vi "TempMonitor.vi"() -> (1 "Temp Out of Range":bool, 3 "Waveform Chart":waveform(dbl)(graph))   [LabVIEW 2013]
panel:
  in  "Min Temp":dbl=15.0
  in  "Max Temp":dbl=30.0
  out "Ch32":dbl
  out "Ch31":dbl
  out "Ch30":dbl
  out "Ch29":dbl
  out "Ch28":dbl
  out "Ch27":dbl
  out "Ch26":dbl
  out "Ch25":dbl
  out "Ch24":dbl
  out "Ch23":dbl
  out "Ch22":dbl
  out "Ch21":dbl
  out "Ch20":dbl
  out "Ch19":dbl
  out "Ch18":dbl
  out "Ch17":dbl
  in  "stop":bool
  out "Ch16":dbl
  out "Ch15":dbl
  out "Ch14":dbl
  out "Ch13":dbl
  out "Ch12":dbl
  out "Ch11":dbl
  out "Ch10":dbl
  out "Ch9":dbl
  out "Ch8":dbl
  out "Ch7":dbl
  out "Ch6":dbl
  out "Ch5":dbl
  out "Ch4":dbl
  out "Ch3":dbl
  out "Ch2":dbl
  out "Ch1":dbl
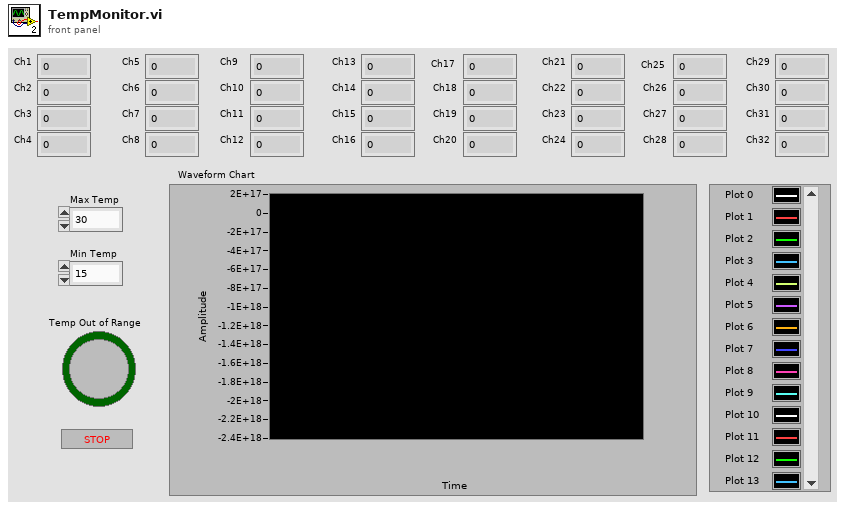
[diagram p1: front panel]
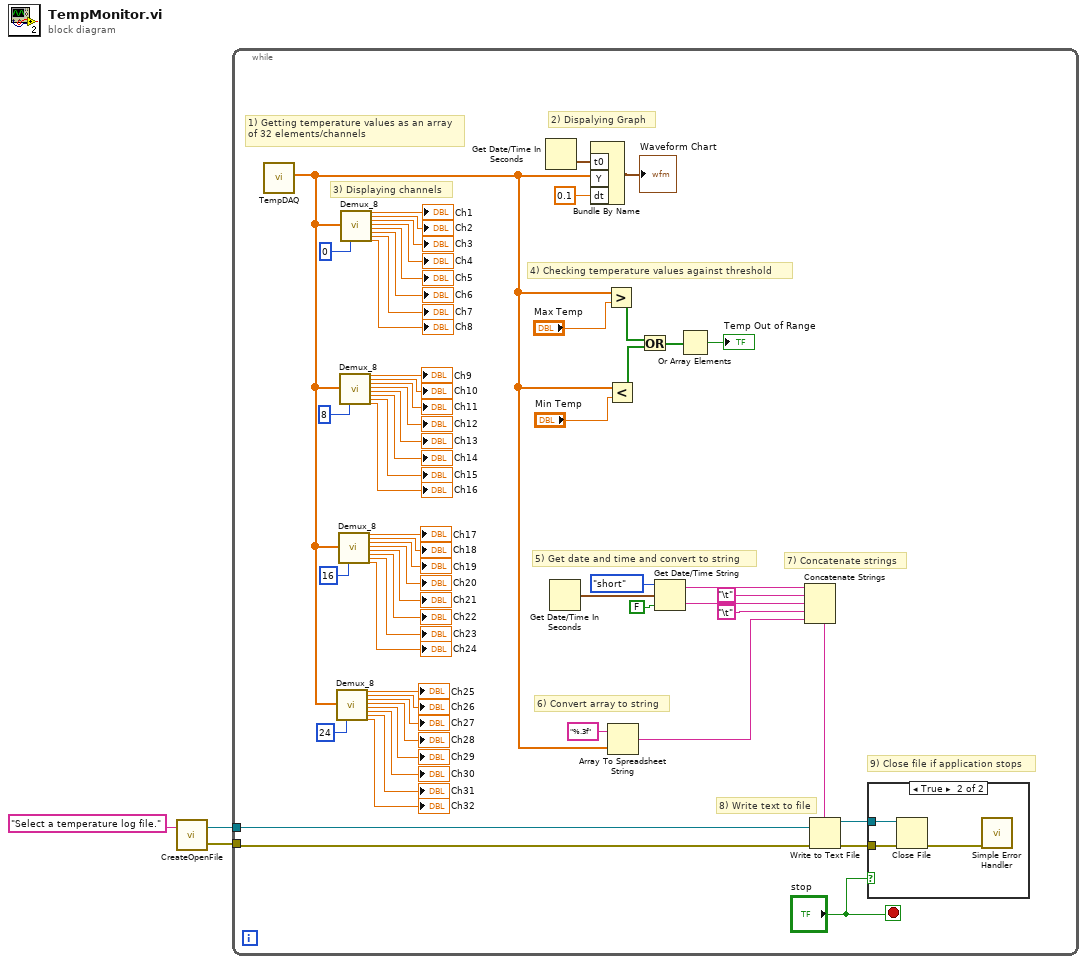
[diagram p0: block diagram]
diagram:
  n1 = call "CreateOpenFile.vi"("Prompt String"="Select a temperature log file.") -> ("error out"=w1:errorcluster, "refnum out"=w2:refnum<file>)  [unwired: 1 in]
  n2 = while {
    tunnel: w2 -> [w8]
    tunnel: w1 -> [w7]
    stop <- "stop" stop-if-true
    # "8) Write text to file"
    # "9) Close file if application stops"
    # "7) Concatenate strings"
    # "6) Convert array to string"
    # "5) Get date and time and convert to string"
    # "4) Checking temperature values against threshold"
    # "1) Getting temperature values as an array\nof 32 elements/channels"
    # "3) Displaying channels"
    # "2) Dispalying Graph"
    n3 = call "TempDAQ.vi"() -> ("Array"=w19:dbl[])  [unwired: 11 in]
    n4 = call "Demux_8.vi"("Data_Array"=w19, "Index"=24) -> ("element_1"=→"Ch25":dbl, "element_2"=→"Ch26":dbl, "element_3"=→"Ch27":dbl, "element_4"=→"Ch28":dbl, "element_5"=→"Ch29":dbl, "element_6"=→"Ch30":dbl, "element_7"=→"Ch31":dbl, "element_8"=→"Ch32":dbl)  [unwired: 18 in]
    n5 = call "Demux_8.vi"("Data_Array"=w19, "Index"=16) -> ("element_1"=→"Ch17":dbl, "element_2"=→"Ch18":dbl, "element_3"=→"Ch19":dbl, "element_4"=→"Ch20":dbl, "element_5"=→"Ch21":dbl, "element_6"=→"Ch22":dbl, "element_7"=→"Ch23":dbl, "element_8"=→"Ch24":dbl)  [unwired: 18 in]
    n6 = call "Demux_8.vi"("Data_Array"=w19, "Index"=8) -> ("element_1"=→"Ch9":dbl, "element_2"=→"Ch10":dbl, "element_3"=→"Ch11":dbl, "element_4"=→"Ch12":dbl, "element_5"=→"Ch13":dbl, "element_6"=→"Ch14":dbl, "element_7"=→"Ch15":dbl, "element_8"=→"Ch16":dbl)  [unwired: 18 in]
    n7 = call "Demux_8.vi"("Data_Array"=w19, "Index"=0) -> ("element_1"=→"Ch1":dbl, "element_2"=→"Ch2":dbl, "element_3"=→"Ch3":dbl, "element_4"=→"Ch4":dbl, "element_5"=→"Ch5":dbl, "element_6"=→"Ch6":dbl, "element_7"=→"Ch7":dbl, "element_8"=→"Ch8":dbl)  [unwired: 18 in]
    n8 = Get Date/Time In Seconds() -> (seconds since 1Jan1904=w48:timestamp)
    n9 = Get Date/Time In Seconds() -> (seconds since 1Jan1904=w17:timestamp)
    n10 = Bundle By Name("t0"=w48, "Y"=w19, "dt"=0.1) -> (→"Waveform Chart":waveform(dbl))  [unwired: 1 in]
    n11 = Greater?(x=w19, y="Max Temp") -> (0:w23:bool[])
    n12 = Less?(x=w19, y="Min Temp") -> (x < y?=w22:bool[])
    n13 = Array To Spreadsheet String(array=w19, 3:"%.3f" ("format string")) -> (spreadsheet string=w10:string)  [unwired: 1 in]
    n14 = Or(x=w23, y=w22) -> (x .or. y?=w21:bool[])
    n15 = Get Date/Time String(date format (0)=enum16{"short", "long", "abbreviated"}."short", seconds (now)=w17, want seconds? (F)=FALSE) -> (date string=w14:string, time string=w12:string)
    n16 = Or Array Elements(Boolean array=w21) -> (logical OR=→"Temp Out of Range":bool)
    n17 = Concatenate Strings(w14, "\t", w12, "\t", w10) -> (w9:string)
    n18 = Write to Text File(file (use dialog)=w8, text=w9, error in=w7) -> (refnum out=w6:refnum<file>, error out=w5:errorcluster)  [unwired: 1 in, 1 out]
    n19 = case shown="True" "stop" {
      tunnel: w6 -> [_ w67]
      tunnel: w5 -> [_ w66]
      frame False {
      }
      frame True {
        n20 = Close File(refnum=w67, error in=w66) -> (error out=w65:errorcluster)  [unwired: 1 out]
        n21 = call <vilib>:"Simple Error Handler.vi"("error in (no error)"=w65) -> ()  [unwired: 4 in, 5 out]
      }
    }
  }
